vi "Initialize Sessions - 1Sess.vi"(6 "initialize and close session behavior":T1, 7 "option string":string, 8 "error in":errorcluster, 9 "reset":bool, 11 "session reservation in":refnum<class "Session Reservation.lvclass">) -> (0 "error out":errorcluster, 1 "channel list":string, 2 "session":refnum<k15>, 3 "session reservation out":refnum<class "Session Reservation.lvclass">)   [LabVIEW 2020, in "niFGEN Sessions.lvlib"]
doc: "Create the NI-FGEN driver session from the <b>session reservation in</b>. Returns an error if more than one NI-FGEN session has been reserved. Use \"Create Session - NSess.vi\" for multiple sessions."
uses:
  niFGEN Sessions.lvlib
  7f77feb2-d2b5-4acd-8f0f-f1b24b7d1641.vi
  Session Factory/Session Factory.lvclass
  APIs/Session Management V1/Session Reservation/Session Reservation.lvclass
  APIs/Session Management V1/Session Reservation/Initialize and Close Session Behavior.ctl
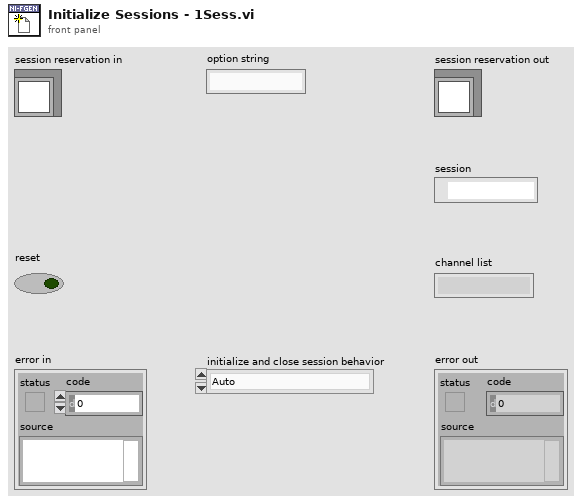
[diagram p1: front panel]
types:
  T1 = typedef "Plug-In SDK Session Management V1 API.lvlib/Session Reservation.lvclass/Initialize and Close Session Behavior.ctl" = enum16{"Auto", "Initialize and Close", "Attach and Detach", "Initialize and Detach", "Attach and Close"}
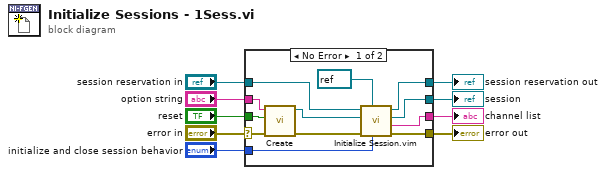
[diagram p0: block diagram]
diagram:
  n1 = case shown="No Error" "error in" {
    selector: "error in" -> [w20 w23]
    tunnel: [w17 w23] -> w8
    tunnel: [w21 w22] -> w6
    tunnel: "session reservation in" -> [w13 w22]
    tunnel: "option string" -> [w18 _]
    tunnel: "reset" -> [w19 _]
    tunnel: [w16 _] -> w3
    tunnel: [w15 _] -> w2
    tunnel: "initialize and close session behavior" -> [w10 _]
    frame No Error {
      n2 = call "Create.vi"("error in"=w20, "reset"=w19, "option string"=w18) -> ("error out"=w12:errorcluster, "session factory out"=w14:refnum<class "Session Factory.lvclass">)  [unwired: 7 in]
      n3 = call "Initialize Session.vim"("initialize and close session behavior"=w10, "session type"=refnum<k15> refnum ("Instrument Handle Out"), "error in"=w12, "session factory"=w14, "session reservation in"=w13) -> ("error out"=w17:errorcluster, "channel list"=w16:string, "session"=w15:refnum<k15>, "session reservation out"=w21:refnum<class "Session Reservation.lvclass">)  [unwired: 3 in]
    }
    frame Error {
    }
  }
  "error out" <- w8
  "session reservation out" <- w6
  "session" <- w2
  "channel list" <- w3
